vi "XML getApiDataValues.vi"(0 "Double in":dbl[](array[numeric]), 1 "XML Data":string, 5 "Integer in":i32[](array[numeric]), 7 "Boolean in":bool[](array[boolean]), 9 "String in":string[](array[string]), 11 "Sample in":T1[](array[typedef])) -> (4 "Double out":dbl[](array[numeric]), 6 "Integer out":i32[](array[numeric]), 8 "Boolean out":bool[](array[boolean]), 10 "String out":string[](array[string]), 15 "Sample out":T1[](array[typedef]))   [LabVIEW 2011]
uses:
  Controls/PIM.API.DataTypes.ctl
  Controls/PIM.API.Response.Samples.ctl
  iQA Sweep Behavior.ctl
  OpenG/string/string.llb/To Proper Case (String)__ogtk.vi
panel:
  in  "Enum (used only for its typeDef info)":T3
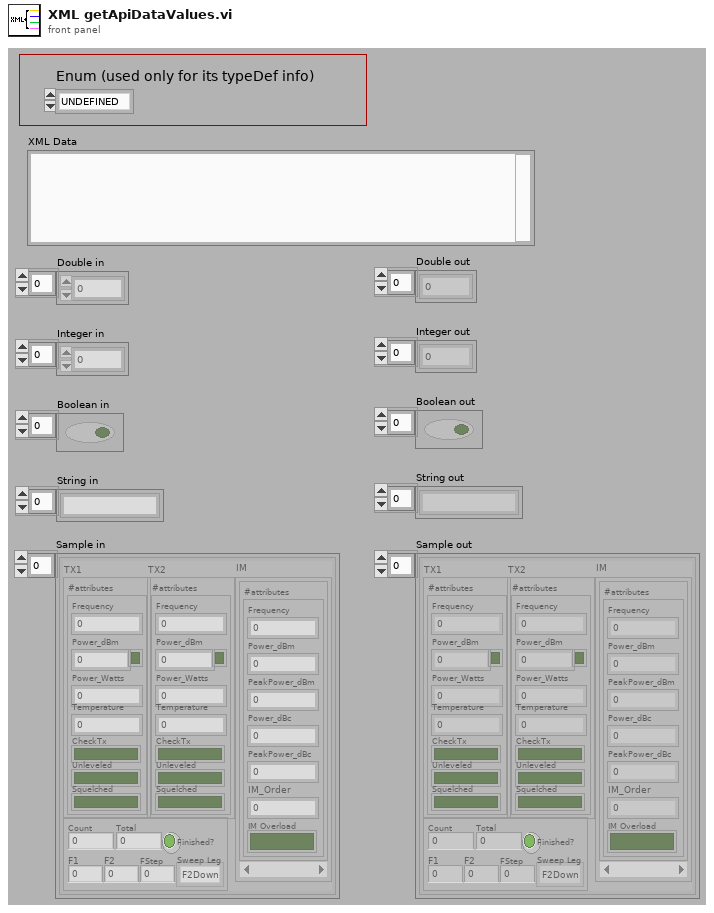
[diagram p1: front panel]
types:
  T1 = typedef "PIM.API.Response.Samples.ctl" = cluster{"TX1":cluster{"#attributes":cluster{"Frequency":dbl, "Power_dBm":dbl, "Power_Watts":dbl, "CheckTx":bool, "Unleveled":bool, "Squelched":bool, "Temperature":dbl, "ToneOn":bool}}, "TX2":cluster{"#attributes":cluster{"Frequency":dbl, "Power_dBm":dbl, "Power_Watts":dbl, "CheckTx":bool, "Unleveled":bool, "Squelched":bool, "Temperature":dbl, "ToneOn":bool}}, "IM":cluster{"#attributes":cluster{"Frequency":dbl, "Power_dBm":dbl, "PeakPower_dBm":dbl, "Power_dBc":dbl, "PeakPower_dBc":dbl, "IM_Order":u8, "IM Overload":bool}}[], "#attributes":cluster{"Count":u32, "Total":u32, "Finished?":bool, "Sweep Leg":T2, "F1":dbl, "F2":dbl, "FStep":dbl}}
  T2 = typedef "iQA Sweep Behavior.ctl" = enum16{"F2Down", "F1Up", "RxMultiIM"}
  T3 = typedef "PIM.API.DataTypes.ctl" = enum16{"UNDEFINED", "double", "integer", "boolean", "string", "sample"}
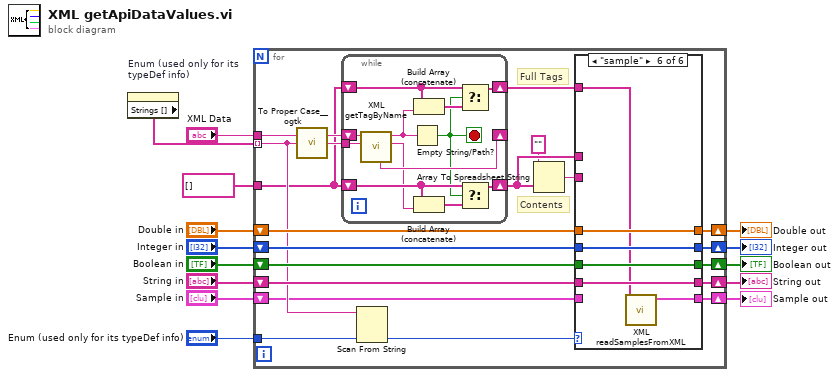
[diagram p0: block diagram]
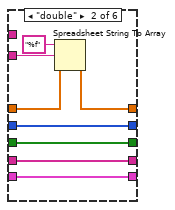
[diagram p3: hidden frame]
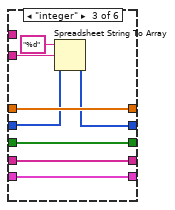
[diagram p4: hidden frame]
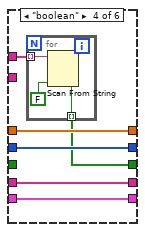
[diagram p5: hidden frame]
diagram:
  n1 = property on="Enum (used only for its typeDef info)" class="Enum (strict)"() -> ("Strings []"=w3:string[])  [unwired: 2 in, 2 out]
  n2 = for {
    tunnel: w3 -> [w19] mode=indexing
    tunnel: "XML Data" -> [w34]
    shift-right: [w28] -> w10
    shift-left: "Double in" -> [w33]
    shift-right: [w27] -> w11
    shift-left: "Integer in" -> [w32]
    shift-right: [w26] -> w12
    shift-left: "Boolean in" -> [w31]
    shift-right: [w25] -> w13
    shift-left: "String in" -> [w30]
    tunnel: string[] [] -> [w16]
    tunnel: "Enum (used only for its typeDef info)" -> [w22]
    shift-right: [w17] -> w1
    shift-left: "Sample in" -> [w18]
    # "Full Tags"
    # "Contents"
    n3 = call-poly "To Proper Case__ogtk.vi"("string"=w19) -> ("proper case string"=w20:string)  [unwired: 4 in]
    n4 = while {
      tunnel: w20 -> [w86]
      shift-right: [w84] -> w24
      shift-left: w16 -> [w83]
      shift-right: [w85] -> _
      shift-left: w34 -> [w87]
      shift-right: [w78] -> w15
      shift-left: w16 -> [w79]
      stop <- w76 stop-if-true
      n5 = call "XML getTagByName.vi"("Tag Name"=w86, "XML String"=w87) -> ("Tag Contents"=w82:string, "Matching Tag"=w77:string, "After Tag"=w85:string)  [unwired: 5 in, 2 out]
      n6 = Empty String/Path?(string/path=w77) -> (empty?=w76:bool)
      n7 = Build Array (concatenate)(w79, w77) -> (w80:string[])
      n8 = Build Array (concatenate)(w83, w82) -> (w81:string[])
      n9 = Select(t=w79, s=w76, f=w80) -> (s? t:f=w78:string[])
      n10 = Select(t=w83, s=w76, f=w81) -> (s? t:f=w84:string[])
    }
    n11 = Scan From String(input string=w19, default 1=w22) -> (output 1=w21:T3)  [unwired: 3 in, 3 out]
    n12 = Array To Spreadsheet String(array=w24, 3:"" ("format string")) -> (spreadsheet string=w29:string)  [unwired: 1 in]
    n13 = case shown="\"sample\"" w21 {
      tunnel: w33 -> [w39 w47 w54 w61 w69 w72]
      tunnel: w32 -> [w38 w44 w53 w59 w67 w73]
      tunnel: w31 -> [w37 w43 w51 _ w68 w74]
      tunnel: w30 -> [w36 w42 w50 w60 _ w75]
      tunnel: w29 -> [_ w46 w55 _ _ _]
      tunnel: [w39 w45 w54 w61 w69 w72] -> w28
      tunnel: [w38 w44 w52 w59 w67 w73] -> w27
      tunnel: [w37 w43 w51 w57 w68 w74] -> w26
      tunnel: [w36 w42 w50 w60 w66 w75] -> w25
      tunnel: w24 -> [_ _ _ w58 w66 _]
      tunnel: w18 -> [w35 w40 w48 w56 w65 _]
      tunnel: [w35 w40 w48 w56 w65 w71] -> w17
      tunnel: w15 -> [_ _ _ _ _ w70]
      frame "UNDEFINED", Default {
      }
      frame "double" {
        n14 = Spreadsheet String To Array(format string="%f", spreadsheet string=w46, array type (2D Dbl)=w47) -> (array=w45:dbl[])  [unwired: 1 in]
      }
      frame "integer" {
        n15 = Spreadsheet String To Array(format string="%d", spreadsheet string=w55, array type (2D Dbl)=w53) -> (array=w52:i32[])  [unwired: 1 in]
      }
      frame "boolean" {
        n16 = for {
          tunnel: w58 -> [w64] mode=indexing
          tunnel: [w62] -> w57 mode=indexing
          n17 = Scan From String(input string=w64, default 1=FALSE) -> (output 1=w62:bool)  [unwired: 3 in, 3 out]
        }
      }
      frame "string" {
      }
      frame "sample" {
        n18 = call "XML readSamplesFromXML.vi"("Samples (XML)"=w70) -> ("Sample"=w71:T1[])  [unwired: 10 in]
      }
    }
  }
  "String out" <- w13
  "Boolean out" <- w12
  "Integer out" <- w11
  "Double out" <- w10
  "Sample out" <- w1
